vi "Get Linker Errors.vi"(8 "error in (no error)":errorcluster, 11 "PPL in":refnum<class "NI_AB_API_DPPL.lvclass">) -> (0 "error out":errorcluster, 2 "Missing VIs Call Chain":variant, 3 "PPL out":refnum<class "NI_AB_API_DPPL.lvclass">, 5 "Has errors?":bool)   [LabVIEW 2020, in "NI_AB_API_DPPL.lvclass"]
uses:
  <vilib>/AppBuilder/AB_API/DPPL/NI_AB_API_DPPL.lvclass
  <vilib>/AppBuilder/AB_API/PPL/NI_AB_API_PPL.lvclass
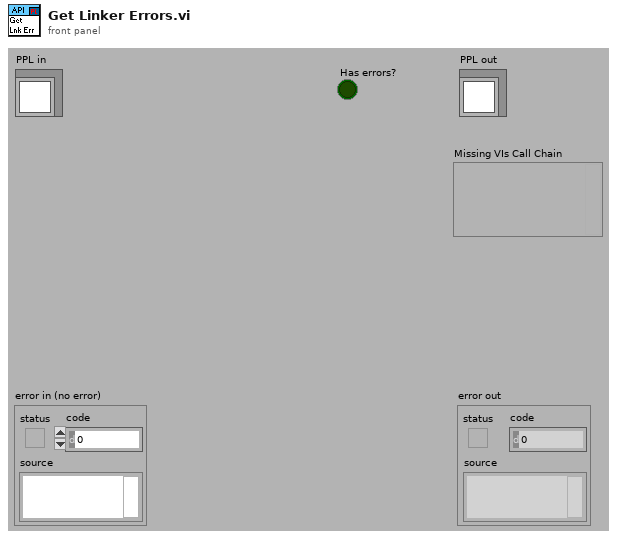
[diagram p1: front panel]
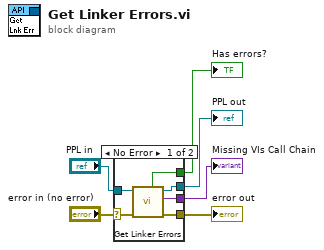
[diagram p0: block diagram]
diagram:
  n1 = case shown="No Error" "error in (no error)" {
    selector: "error in (no error)" -> [w7 w14]
    tunnel: [w8 w14] -> w5
    tunnel: [w11 w13] -> w3
    tunnel: "PPL in" -> [w12 w13]
    tunnel: [w10 _] -> w2
    tunnel: [w9 _] -> w1
    frame No Error {
      n2 = call-parent "Get Linker Errors.vi"("error in (no error)"=w7, "PPL in"=w12) -> ("error out"=w8:errorcluster, "Missing VIs Call Chain"=w9:variant, "PPL out"=w11:refnum<class "NI_AB_API_DPPL.lvclass">, "Has errors?"=w10:bool)  [unwired: 6 in]
    }
    frame Error {
    }
  }
  "error out" <- w5
  "PPL out" <- w3
  "Has errors?" <- w2
  "Missing VIs Call Chain" <- w1
